vi "DFF.vi"(1 "Clock":bool, 3 "Input":bool) -> (0 "Output":bool)   [LabVIEW 2020, in "Hack.lvlib"]
uses:
  Hack.lvlib
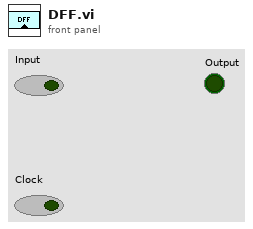
[diagram p1: front panel]
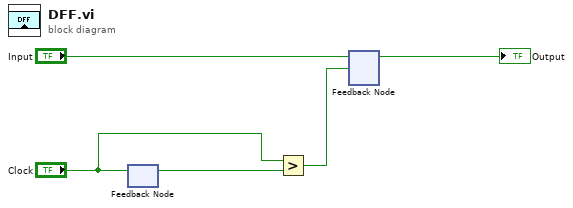
[diagram p0: block diagram]
diagram:
  n1 = feedback #1() -> (w3:bool)  [unwired: 1 in]
  n2 = feedback-in #1("Clock") -> ()
  n3 = Greater?(x="Clock", y=w3) -> (0:w2:bool)
  n4 = feedback-in #2("Input", w2) -> ()
  n5 = feedback #2() -> (→"Output":bool)  [unwired: 1 in]
